vi "主VI.vi"() -> ()   [LabVIEW 2016]
uses:
  <vilib>/MGI/Panel Manager/Panel/Panel/Window/Window.lvclass
  C:/Program Files (x86)/National Instruments/LabVIEW 2016/vi.lib/MGI/Panel Manager/Panel/Panel/Panel.lvclass
  <vilib>/MGI/Panel Manager/Panel/Panel/Window/Window.vi
  <vilib>/MGI/Panel Manager/Panel/Panel.lvlib
panel:
  out "运行信息":string
  in  "查看":bool
  in  "关闭所有任务":bool
  in  "已有任务":u16(ring) items=["ABC", "ABCD"]
  in  "新建":bool
  in  "新建任务名":string
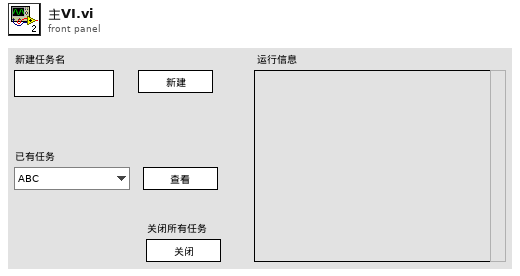
[diagram p1: front panel]
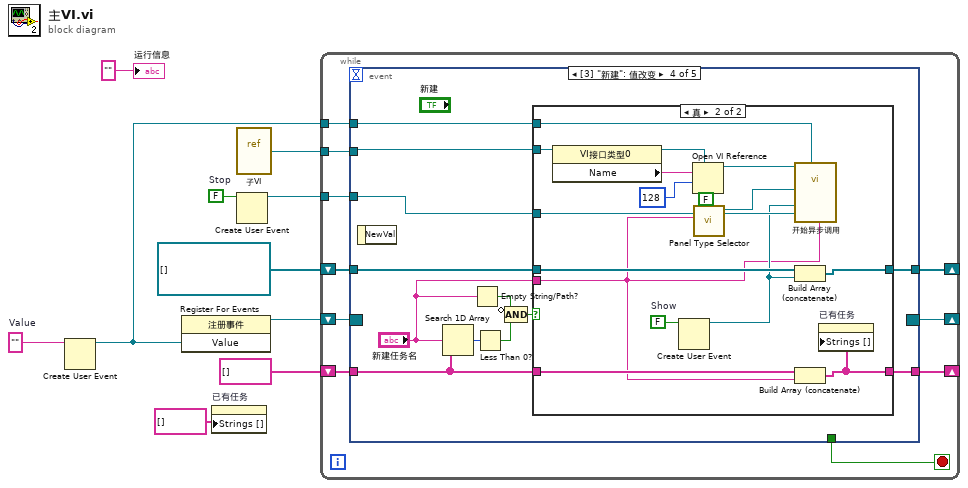
[diagram p0: block diagram]
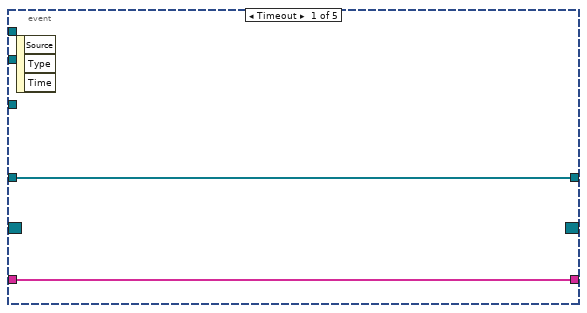
[diagram p2: hidden frame]
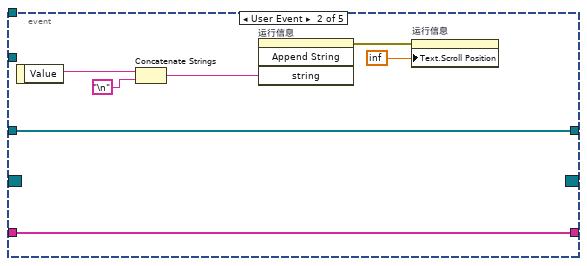
[diagram p3: hidden frame]
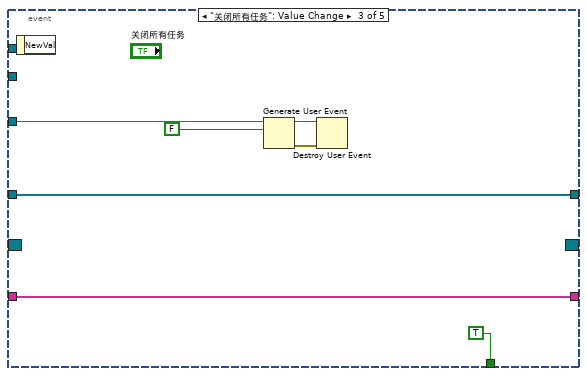
[diagram p4: hidden frame]
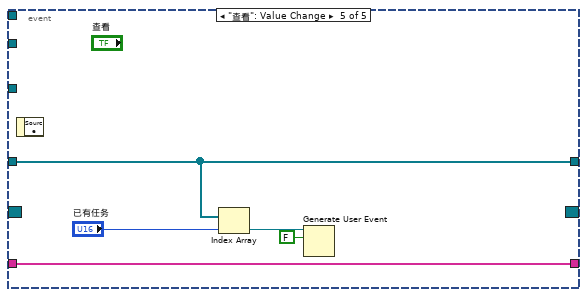
[diagram p6: hidden frame]
diagram:
  w9 = ""  # Value
  w10 = FALSE  # Stop
  n1 = Create User Event(user event datatype=w9) -> (user event=w3:refnum<user-event>)  [unwired: 1 in, 1 out]
  n2 = register-events(w3) -> (reference out=w8:refnum<event-registration>)  [unwired: 2 in, 1 out]
  n3 = property on="已有任务" class="Ring (严格)"("Strings []"=string[] []) -> ()  [unwired: 2 in, 2 out]
  n4 = vi-ref "子VI.vi"() -> (w5:refnum<vi>)
  n5 = Create User Event(user event datatype=w10) -> (user event=w6:refnum<user-event>)  [unwired: 1 in, 1 out]
  n6 = while {
    shift-right: [w19] -> _
    shift-left: w8 -> [w20]
    shift-right: [w17] -> _
    shift-left: refnum<user-event>[] [] ("Show") -> [w18]
    tunnel: w6 -> [w16]
    tunnel: w5 -> [w15]
    shift-right: [w13] -> _
    shift-left: string[] [] -> [w14]
    tunnel: w3 -> [w12]
    stop <- w11 stop-if-true
    n7 = event shown="[3] \"新建\": 值改变" {
      selector: w20 -> [_ _ _ _ _]
      dyn-events: [_ _ _ _ _] -> w19
      timeout: _ -> [_ _ _ _ _]
      tunnel: w18 -> [w22 w29 w30 w45 w70]
      tunnel: [w22 w29 w30 w44 w70] -> w17
      tunnel: w16 -> [_ _ w36 w47 _]
      tunnel: w15 -> [_ _ _ w48 _]
      tunnel: w14 -> [w21 w28 w32 w39 w71]
      tunnel: [w21 w28 w32 w38 w71] -> w13
      tunnel: w12 -> [_ _ _ w43 _]
      tunnel: [_ _ TRUE _ _] -> w11
      event Timeout {
        n8 = event-data() -> ()  [unwired: 1 in, 3 out]
      }
      event User Event {
        n9 = event-data() -> ("Value"=w27:string)  [unwired: 1 in]
        n10 = Concatenate Strings(w27, "\n") -> (w25:string)
        n11 = invoke on="运行信息" class="Str" method="Append String"("string"=w25) -> (error out=w24:errorcluster)  [unwired: 3 in, 3 out]
        n12 = property on="运行信息" class="Str"(error in=w24, "Text.Scroll Position"=inf) -> ()  [unwired: 1 in, 2 out]
      }
      event "关闭所有任务": Value Change {
        n13 = event-data() -> ()  [unwired: 1 in, 1 out]
        n14 = Generate User Event(user event=w36, event data cluster=FALSE ("事件数据")) -> (user event out=w34:refnum<user-event>, error out=w35:errorcluster)  [unwired: 2 in]
        n15 = Destroy User Event(user event=w34, error in=w35) -> ()  [unwired: 1 out]
      }
      event "新建": Value Change {
        n16 = event-data() -> ()  [unwired: 1 in, 1 out]
        n17 = Search 1D Array(1D array=w39, element="新建任务名") -> (index of element=w46:i32)  [unwired: 1 in]
        n18 = Empty String/Path?(string/path="新建任务名") -> (empty?=w42:bool)
        n19 = Less Than 0?(x=w46) -> (x < 0?=w41:bool)
        n20 = Compound Arithmetic op=AND ("复合运算")(invert w42, w41) -> (w40:bool)
        n21 = case shown="真" w40 {
          tunnel: w48 -> [_ w66]
          tunnel: w47 -> [_ w59]
          tunnel: w45 -> [w50 w57]
          tunnel: [w50 w56] -> w44
          tunnel: w43 -> [_ w54]
          tunnel: w39 -> [w49 w53]
          tunnel: [w49 w52] -> w38
          tunnel: "新建任务名" -> [_ w51]
          frame False {
          }
          frame True {
            w60 = FALSE  # Show
            n22 = property class="VI接口类型0"(reference=w66) -> (reference out=w64:refnum<vi>, "Name"=w65:string)  [unwired: 1 in, 1 out]
            n23 = Create User Event(user event datatype=w60) -> (user event=w55:refnum<user-event>)  [unwired: 1 in, 1 out]
            n24 = Open VI Reference(type specifier VI Refnum (for type only)=w64, vi path=w65, options=128 ("选项")) -> (vi reference=w62:refnum<vi>)  [unwired: 3 in, 1 out]
            n25 = call-poly <vilib>:"Panel Type Selector.vi"("Autoshow? (T)"=FALSE, "Default Title"=w51) -> ("Window out"=w61:refnum<class "Window.lvclass">)  [unwired: 8 in, 1 out]
            n26 = call-by-ref "开始异步调用"(reference=w62, "ID"=w51, "Value"=w54, "Stop"=w59, "Show"=w55, "Panel"=w61) -> ()  [unwired: 8 in, 2 out]
            n27 = Build Array (concatenate)(w57, w55) -> (w56:refnum<user-event>[])
            n28 = Build Array (concatenate)(w53, w51) -> (w52:string[])
            n29 = property on="已有任务" class="Ring (严格)"("Strings []"=w52) -> ()  [unwired: 2 in, 2 out]
          }
        }
      }
      event "查看": Value Change {
        n30 = event-data() -> ()  [unwired: 1 in, 1 out]
        n31 = Index Array(array=w70, index="已有任务") -> (element=w68:refnum<user-event>)
        n32 = Generate User Event(user event=w68, event data cluster=FALSE ("事件数据")) -> ()  [unwired: 2 in, 2 out]
      }
    }
  }
  "运行信息" <- ""
